vi "Write Holding Registers.vi"(6 "Ignore Mask?":bool=TRUE, 7 "Regs to Write":bool[](array[boolean]), 8 "error in (no error)":errorcluster, 9 "Channel Data":T1[](array[typedef]), 10 "Values":dbl[](array[numeric]), 11 "Modbus API.lvlibp:Modbus API":refnum<class "Modbus Master.lvclass">) -> (0 "error out":errorcluster)   [LabVIEW 2020, in "Modbus Master Engine.lvlib"]
uses:
  Modbus Master Engine.lvlib
  Custom Device/Shared/Controls/Data Model/Channel.ctl
  Custom Device/System Explorer/SubVIs/Modbus Type.ctl
  <vilib>/NI VeriStand/Custom Device API/Custom Device Channel Type.ctl
  Custom Device/Shared/Controls/Data Model/Mapping.ctl
  Custom Device/Shared/Controls/Data Model/DataType.ctl
  <vilib>/NI VeriStand/Custom Device API/Custom Device Item Ref.ctl
  API/Master/Modbus Master.lvclass
  Custom Device/Shared/Modbus Master Shared.lvlib
  <vilib>/NI VeriStand/Custom Device API/Custom Device API.lvlib
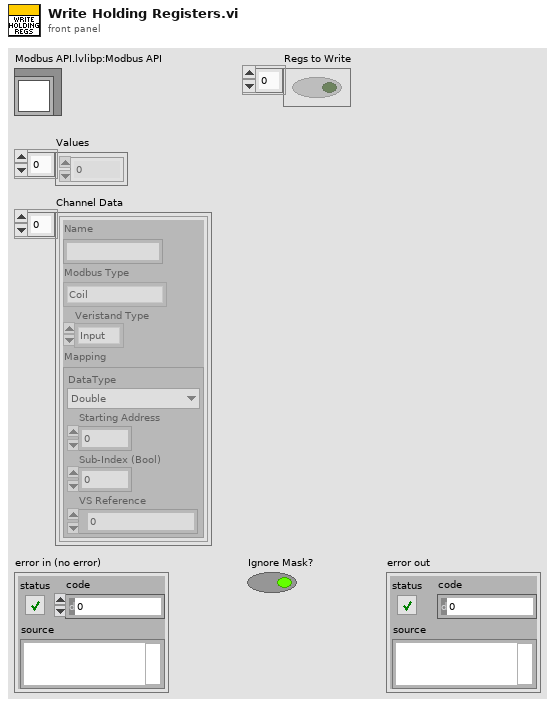
[diagram p1: front panel]
types:
  T1 = typedef "Modbus Master Shared.lvlib/Channel.ctl" = cluster{"Name":string, "Modbus Type":T2, "Veristand Type":T3, "Mapping":T4}
  T2 = typedef "Modbus Master Shared.lvlib/Modbus Type.ctl" = enum16{"Coil", "Discrete Input", "Holding Register", "Input Register"}
  T3 = typedef "Custom Device API.lvlib/Custom Device Channel Type.ctl" = enum16{"Input", "Output"}
  T4 = typedef "Modbus Master Shared.lvlib/Mapping.ctl" = cluster{"DataType":T5, "Starting Address":u16, "Sub-Index (Bool)":u16, "VS Reference":T6}
  T5 = typedef "Modbus Master Shared.lvlib/DataType.ctl" = enum16{"Double", "Single", "I64", "I32", "I16", "I8", "U64", "U32", "U16", "U8", "Boolean"}
  T6 = typedef "Custom Device API.lvlib/Custom Device Item Ref.ctl" = u64
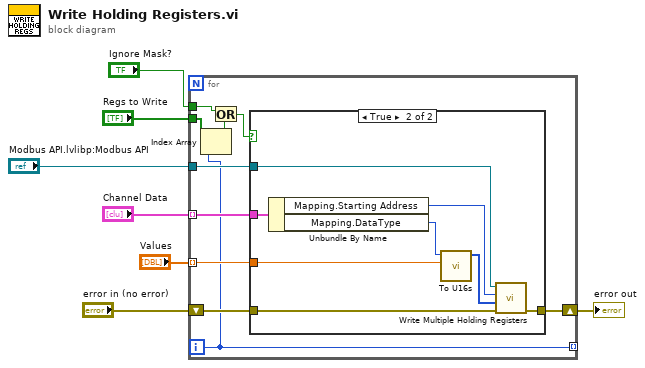
[diagram p0: block diagram]
diagram:
  n1 = for {
    tunnel: "Modbus API.lvlibp:Modbus API" -> [w17]
    tunnel: "Values" -> [w14] mode=indexing
    shift-right: [w15] -> w4
    shift-left: "error in (no error)" -> [w16]
    tunnel: "Regs to Write" -> [w12]
    tunnel: "Channel Data" -> [w13] mode=indexing
    tunnel: "Ignore Mask?" -> [w11]
    tunnel: [w8] -> _ mode=indexing
    i -> [w8]
    n2 = Index Array(array=w12, index=w8) -> (element=w9:bool)
    n3 = Or(x=w11, y=w9) -> (x .or. y?=w10:bool)
    n4 = case shown="True" w10 {
      tunnel: w17 -> [_ w21]
      tunnel: w16 -> [w18 w23]
      tunnel: [w18 w24] -> w15
      tunnel: w14 -> [_ w19]
      tunnel: w13 -> [_ w26]
      frame False {
      }
      frame True {
        n5 = Unbundle By Name(w26) -> ("Mapping.Starting Address"=w22:u16, "Mapping.DataType"=w25:T5)
        n6 = call "To U16s.vi"("Numeric"=w19, "DataType"=w25) -> ("Array"=w20:u16[])  [unwired: 9 in]
        n7 = call-dynamic "Write Multiple Holding Registers.vi"("error in"=w23, "registers to write"=w20, "starting address"=w22, "Modbus master in"=w21) -> ("error out"=w24:errorcluster)  [unwired: 6 in, 1 out]
      }
    }
  }
  "error out" <- w4
